vi "I2C_to_Target_Spec.vi"(0 "I2C_Data":T1={"Vmin"=0.0, "Vmax"=1.0, "Input"="", "Off_Set (uS)"=0.0, "T_HD_STA (uS)"=0.0, "Sample_Per_Us"=0.0, "T_HD_DAT (uS)"=0.0, "T_SU_DAT (uS)"=0.0, "Frequency (kHz)"=0.0, "T_SU_STO"=0.0, "T_Off (uS)"=0.0, "T_On (uS)"=0.0, "T_BUF"=0.0, "Target_Address"=0, "Selected_Register_Address"=0, "Byte_Array"=[], "Target_Name"="", "Register_Name"=[], "Register_Address"=[], "Target_Type"=0, "Register_Data"=[]} {"Target_Type" items=["10 Bit Address", "7 Bit Address"]; "Selected_Register_Address" format="%x"; "Target_Address" format="%x"}) -> (4 "Target_Specification":T3 {"Target_Address" format="%x"; "Target_Type" items=["10 Bit Address", "7 Bit Address"]; "T_On (uS)" min=1e-06; "T_Off (uS)" min=1e-06})   [LabVIEW 2023]
doc: "Used to convert the I2C data to Target Spec Data"
uses:
  Controls/Add_Target_Specification_.ctl
  Controls/Customized_Ring.ctl
  Controls/I2C_Data.ctl
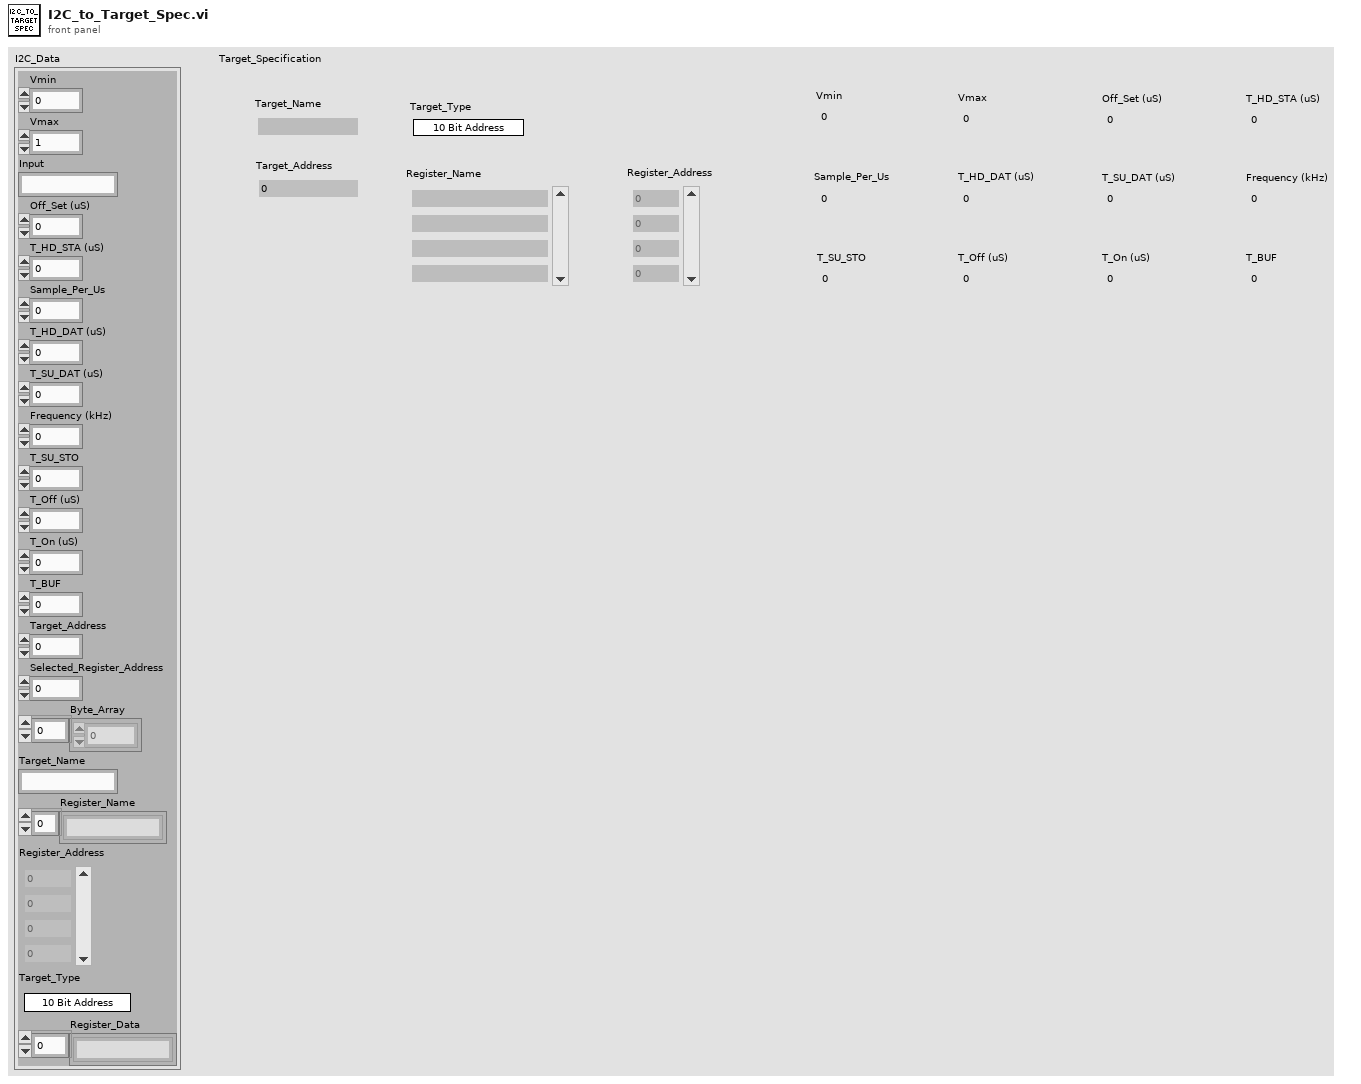
[diagram p1: front panel]
types:
  T1 = typedef "I2C_Data.ctl" = cluster{"Vmin":dbl, "Vmax":dbl, "Input":string, "Off_Set (uS)":dbl, "T_HD_STA (uS)":dbl, "Sample_Per_Us":dbl, "T_HD_DAT (uS)":dbl, "T_SU_DAT (uS)":dbl, "Frequency (kHz)":dbl, "T_SU_STO":dbl, "T_Off (uS)":dbl, "T_On (uS)":dbl, "T_BUF":dbl, "Target_Address":u16, "Selected_Register_Address":u8, "Byte_Array":u8[], "Target_Name":string, "Register_Name":string[], "Register_Address":u8[], "Target_Type":T2, "Register_Data":string[]}
  T2 = typedef "Customized_Ring.ctl" = u16
  T3 = typedef "Add_Target_Specification_.ctl" = cluster{"Target_Name":string, "Register_Name":string[], "Register_Address":u16[], "Vmin":dbl, "Vmax":dbl, "Off_Set (uS)":dbl, "T_HD_STA (uS)":dbl, "T_HD_DAT (uS)":dbl, "T_SU_DAT (uS)":dbl, "Frequency (kHz)":dbl, "T_SU_STO":dbl, "T_Off (uS)":dbl, "T_On (uS)":dbl, "T_BUF":dbl, "Sample_Per_Us":dbl, "Target_Type":T2, "Target_Address":u16}
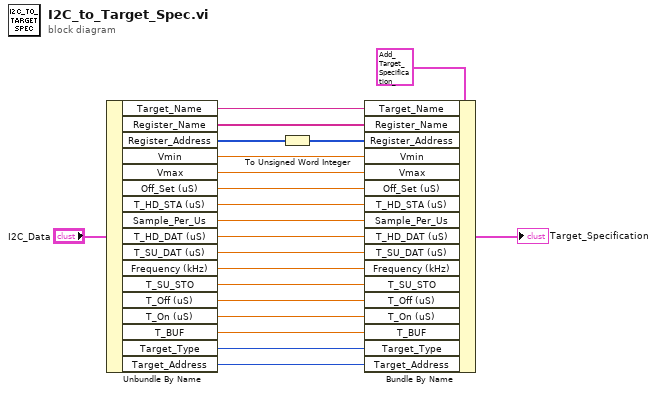
[diagram p0: block diagram]
diagram:
  n1 = Unbundle By Name("I2C_Data") -> ("Target_Name"=w17:string, "Register_Name"=w18:string[], "Register_Address"=w19:u8[], "Vmin"=w5:dbl, "Vmax"=w6:dbl, "Off_Set (uS)"=w7:dbl, "T_HD_STA (uS)"=w8:dbl, "Sample_Per_Us"=w9:dbl, "T_HD_DAT (uS)"=w10:dbl, "T_SU_DAT (uS)"=w11:dbl, "Frequency (kHz)"=w12:dbl, "T_SU_STO"=w13:dbl, "T_Off (uS)"=w14:dbl, "T_On (uS)"=w15:dbl, "T_BUF"=w16:dbl, "Target_Type"=w21:T2, "Target_Address"=w3:u16)
  n2 = To Unsigned Word Integer(number=w19) -> (unsigned 16bit integer=w20:u16[])
  n3 = Bundle By Name(cluster=T3 {"Target_Name"="", "Register_Name"=[], "Register_Address"=[], "Vmin"=0.0, "Vmax"=0.0, "Off_Set (uS)"=0.0, "T_HD_STA (uS)"=0.0, "T_HD_DAT (uS)"=0.0, "T_SU_DAT (uS)"=0.0, "Frequency (kHz)"=0.0, "T_SU_STO"=0.0, "T_Off (uS)"=0.0, "T_On (uS)"=0.0, "T_BUF"=0.0, "Sample_Per_Us"=0.0, "Target_Type"=0, "Target_Address"=0} ("Target_Specification"), "Target_Name"=w17, "Register_Name"=w18, "Register_Address"=w20, "Vmin"=w5, "Vmax"=w6, "Off_Set (uS)"=w7, "T_HD_STA (uS)"=w8, "Sample_Per_Us"=w9, "T_HD_DAT (uS)"=w10, "T_SU_DAT (uS)"=w11, "Frequency (kHz)"=w12, "T_SU_STO"=w13, "T_Off (uS)"=w14, "T_On (uS)"=w15, "T_BUF"=w16, "Target_Type"=w21, "Target_Address"=w3) -> (→"Target_Specification":T3)
